vi "XYWaveform.vi"(11 "XYWaveformIN":waveform(dbl)) -> (3 "XYWaveformOut":waveform(dbl))   [LabVIEW 2018]
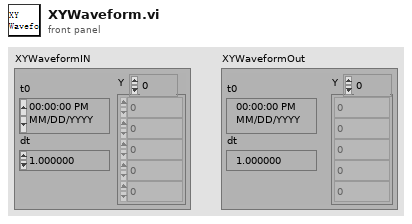
[diagram p1: front panel]
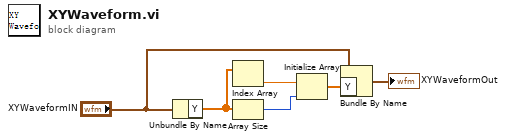
[diagram p0: block diagram]
diagram:
  n1 = Unbundle By Name("XYWaveformIN") -> ("Y"=w3:dbl[])
  n2 = Index Array(array=w3) -> (element=w4:dbl)  [unwired: 1 in]
  n3 = Array Size(array=w3) -> (size(s)=w2:i32)
  n4 = Initialize Array(w4, w2) -> (w1:dbl[])
  n5 = Bundle By Name(cluster="XYWaveformIN", "Y"=w1) -> (→"XYWaveformOut":waveform(dbl))
